vi "3MultAddition.vi"() -> ()   [LabVIEW 2025]
panel:
  out "Meter":dbl(knob) scale=0.0..10.0
  in  "Numeric":dbl
  in  "Dial":dbl(knob) scale=0.0..10.0
  in  "Knob":dbl(knob) scale=0.0..10.0
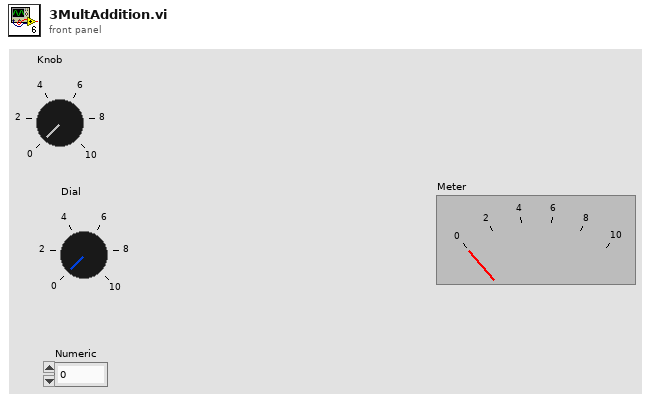
[diagram p1: front panel]
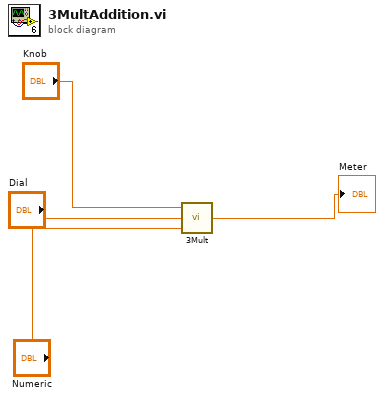
[diagram p0: block diagram]
diagram:
  n1 = call "3Mult.vi"("x3"="Numeric", "x2"="Dial", "x1"="Knob") -> ("Result"=→"Meter":dbl)
